vi "MercuryConfigured.vi"() -> ()   [LabVIEW 2014]
panel:
  out "Mercury Configured?":bool
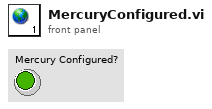
[diagram p1: front panel]
diagram:
